vi "Create Path and Folders.vi"(8 "error in (no error)":errorcluster, 11 "String Path":string) -> (0 "error out":errorcluster, 3 "path for csv file":path)   [LabVIEW 2023, in "WritingDataFile.lvlib"]
uses:
  WritingDataFile.lvlib
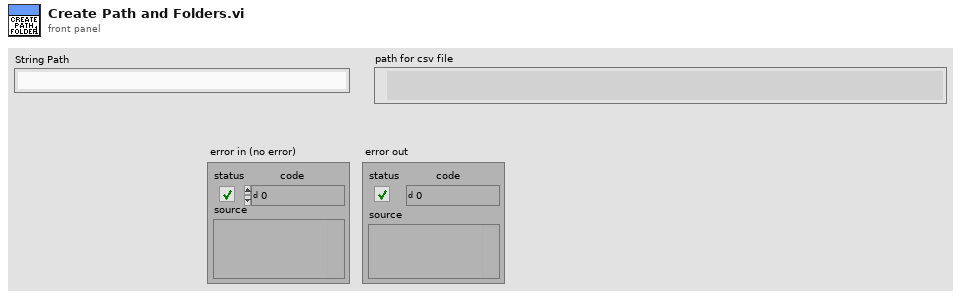
[diagram p1: front panel]
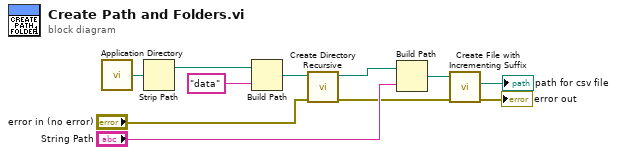
[diagram p0: block diagram]
diagram:
  n1 = call <vilib>:"Application Directory.vi"() -> ("Application Directory"=w8:path)
  n2 = Strip Path(path=w8) -> (stripped path=w10:path)  [unwired: 1 out]
  n3 = Build Path(base path=w10, name or relative path="data") -> (appended path=w6:path)
  n4 = call <vilib>:"Create Directory Recursive.vi"("error in (no error)"="error in (no error)", "directory"=w6) -> ("error out"=w2:errorcluster, "directory copy"=w4:path)  [unwired: 3 in, 1 out]
  n5 = Build Path(base path=w4, name or relative path="String Path") -> (appended path=w3:path)
  n6 = call <vilib>:"Create File with Incrementing Suffix.vi"("error in (no error)"=w2, "file path"=w3) -> ("error out"=→"error out":errorcluster, "actual path"=→"path for csv file":path)  [unwired: 7 in, 1 out]
